vi "System.vi"() -> ()   [LabVIEW 2020]
uses:
  <vilib>/Instr/_visa.llb/VISA Configure Serial Port (Instr).vi
  <vilib>/httpClient/PUTBuffer.vi
  <vilib>/express/express analysis/Spectral/Block/exnSpectralBlock spectral measurements peak poly.vi
  <vilib>/express/express analysis/Spectral/Block/exnSpectralBlock spectral measurements peak DDT.vi
  <vilib>/express/express analysis/Spectral/XNode/ExpressSpectralMeasurementsBlockNode.xnode
  <vilib>/httpClient/LabVIEWHTTPClient.lvlib
panel:
  out "Poor Ventilation":bool
  out "Blade Impact":bool
  out "Normal Operation":bool
  out "?":dbl(knob) scale=0.0..3000.0
  out "Fault 2":dbl
  out "Prediction Started":bool
  out "?":u32
  in  "Current Sensor Threshold":dbl(slide) scale=2.5..2.55
  in  "Arduino COM port":refnum<visa-resource-name>
  out "Vibration Peak":dbl
  out "AI Output":dbl
  out "fft-peak":dbl
  out "data 2":dynamicdata(graph) caption="Sensor Output"
  out "Current Sesnor Output":dbl
  out "?":dbl
  out "?":dbl(knob) scale=0.0..5.0
  out "?":dbl
  out "?":dbl(slide) scale=0.0..100.0
  in  "System stop":bool
  out "?":dbl
  out "FFT":dynamicdata(graph)
  out "Time Domain":dynamicdata(graph)
  # "Fault Detection System For an Industrial Exhaust Fan"
  # "Temperature Sensor"
  # "Current Sensor"
  # "Vibration Sensor"
  # "RPM Sensor"
  # "System Up time (ms)"
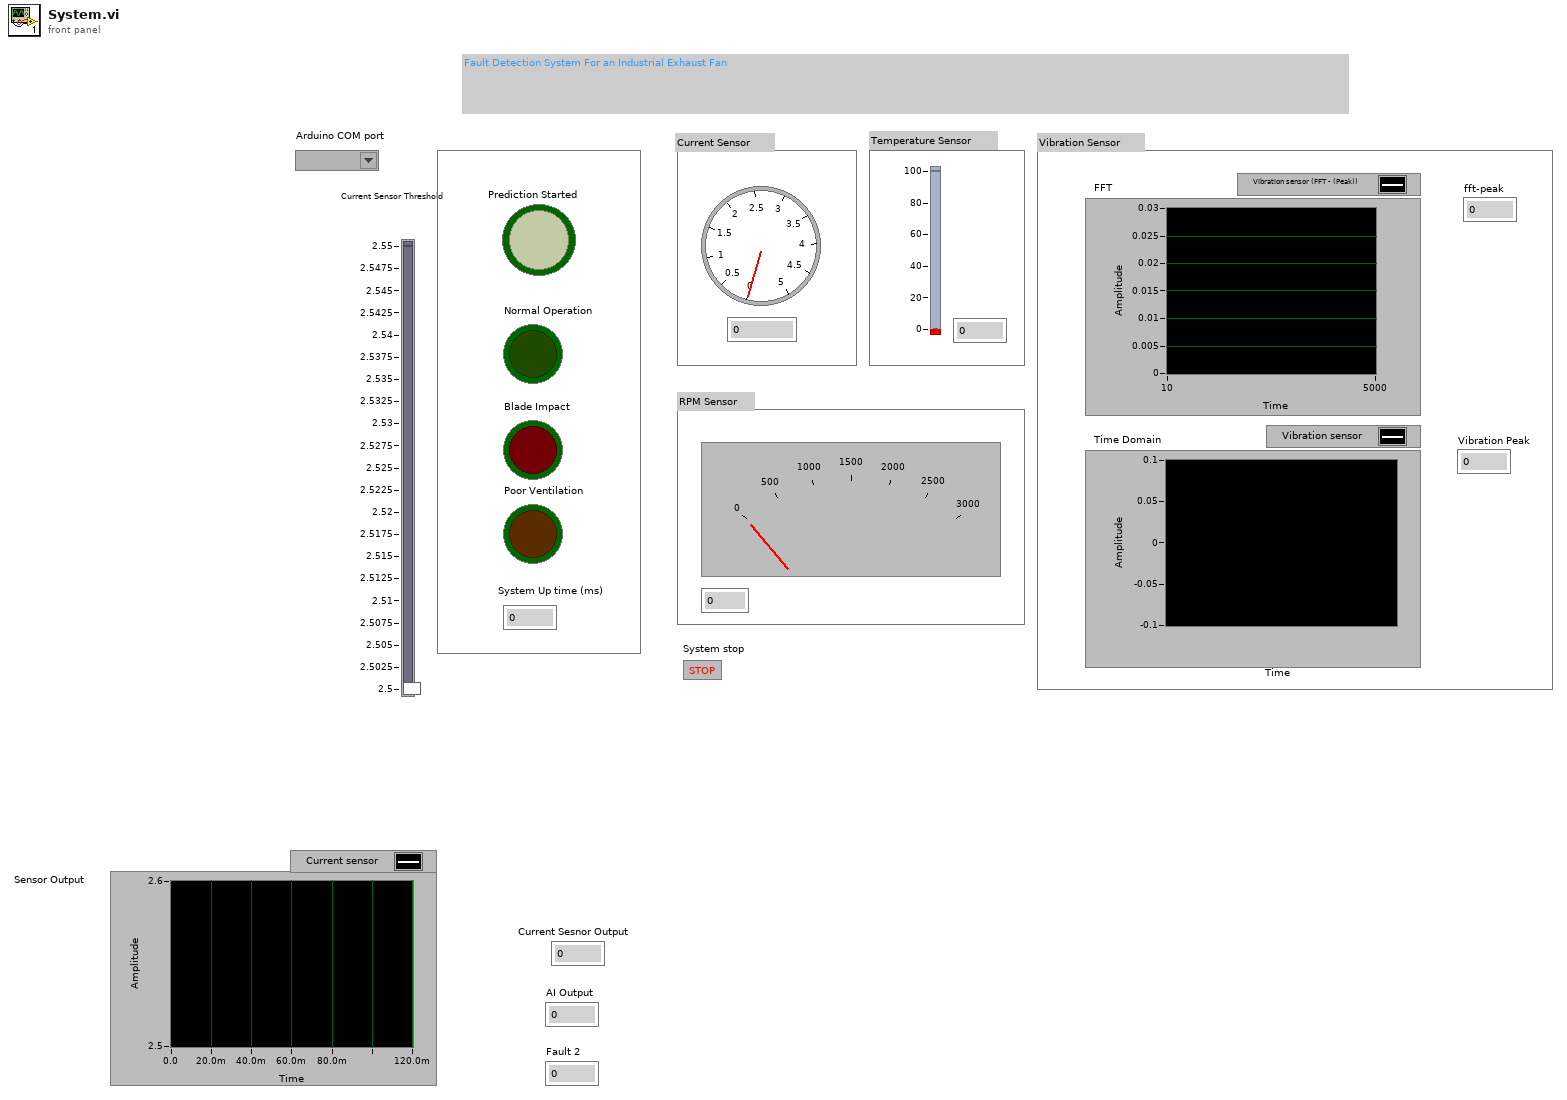
[diagram p1: front panel]
types:
  T1 = cluster{"averaging mode":u16, "weighting mode":u16, "number of averages":u32}
  T2 = cluster{"dB On (F)":bool, "unwrap phase (F)":bool, "convert to degree (F)":bool}
  T3 = typedef "LabVIEWHTTPClient.lvlib/ClientHandle.ctl" = refnum<k1>
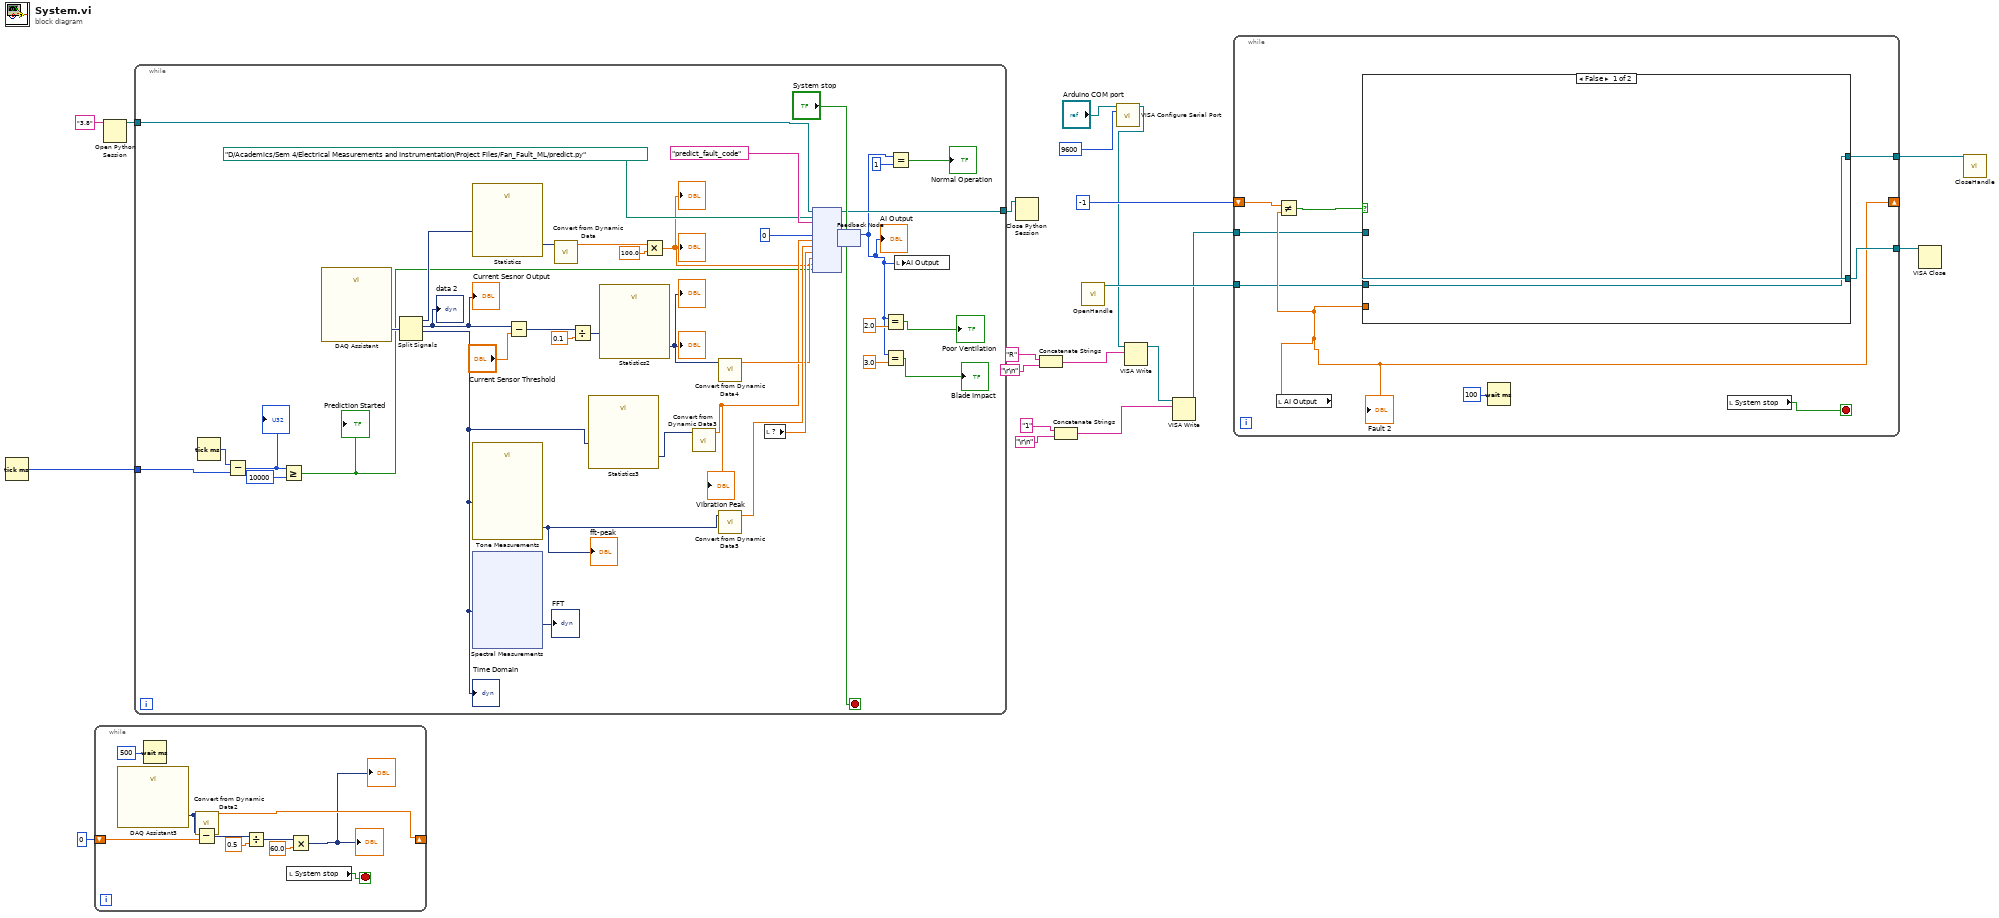
[diagram p0: block diagram]
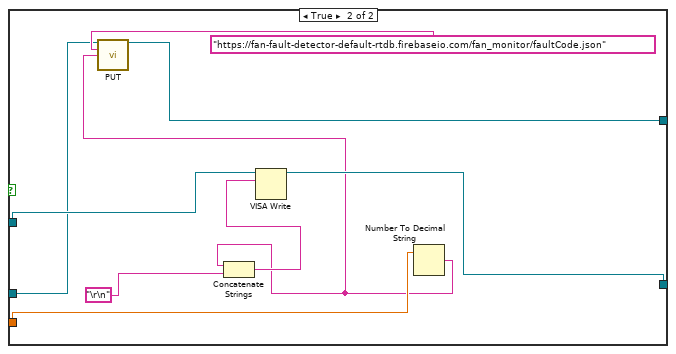
[diagram p2: hidden frame]
diagram:
  n1 = Tick Count (ms)() -> (millisecond timer value=w6:u32)
  n2 = while {
    shift-right: [w28] -> _
    shift-left: 0 -> [w29]
    stop <- w22 stop-if-true
    n3 = call "DAQ Assistant3"() -> ("data"=w23:dynamicdata)  [unwired: 16 in, 3 out]
    n4 = Wait (ms)(milliseconds to wait=u32 500) -> ()  [unwired: 1 out]
    n5 = call "Convert from Dynamic Data2"("Dynamic Data Type"=w23) -> ("Scalar"=w28:dbl)  [unwired: 3 in]
    n6 = Subtract(x=w23, y=w29) -> (x-y=w27:dynamicdata)
    n7 = Divide(x=w27, y=0.5) -> (x/y=w26:dynamicdata)
    n8 = local read "System stop"() -> (w22:bool)
    n9 = Multiply(x=w26, y=60.0) -> (x*y=→"?" →"?":dynamicdata)
  }
  n10 = Open Python Session(python version="3.8" ("Python version")) -> (session out=w18:refnum<k35>)  [unwired: 2 in, 1 out]
  n11 = while {
    tunnel: w18 -> [w51]
    tunnel: [w52] -> w17
    tunnel: w6 -> [w39]
    stop <- "System stop" stop-if-true
    n12 = Tick Count (ms)() -> (millisecond timer value=w42:u32)
    n13 = Subtract(x=w42, y=w39) -> (x-y=w41:u32)
    "?" <- w41
    n14 = Greater Or Equal?(x=w41, y=u32 10000) -> (x >= y?=w38:bool)
    "Prediction Started" <- w38
    n15 = call "DAQ Assistant"() -> ("data"=w63:dynamicdata)  [unwired: 16 in, 3 out]
    n16 = Split Signals(w63) -> (w60:dynamicdata, w62:dynamicdata, w49:dynamicdata)  [unwired: 4 in, 1 out]
    "Time Domain" <- w49
    "Current Sesnor Output" <- w62
    "data 2" <- w62
    n17 = call "Statistics"("Signals"=w60) -> ("Arithmetic Mean"=w68:dynamicdata)  [unwired: 25 in, 1 out]
    n18 = call "Tone Measurements"("Signals"=w49) -> ("Amplitude"=w50:dynamicdata)  [unwired: 8 in, 2 out]
    "fft-peak" <- w50
    n19 = xnode "Spectral Measurements"("Signals"=w49) -> ("FFT - (Peak)"=→"FFT":dynamicdata)  [unwired: 1 in, 2 out]
    n20 = Subtract(x=w62, y="Current Sensor Threshold") -> (x-y=w65:dynamicdata)
    n21 = call "Convert from Dynamic Data"("Dynamic Data Type"=w68) -> ("Scalar"=w67:dbl)  [unwired: 3 in]
    n22 = Divide(x=w65, y=0.1) -> (x/y=w61:dynamicdata)
    n23 = call "Statistics3"("Signals"=w49) -> ("Maximum"=w48:dynamicdata)  [unwired: 25 in, 1 out]
    n24 = call "Statistics2"("Signals"=w61) -> ("Arithmetic Mean"=w59:dynamicdata)  [unwired: 25 in, 1 out]
    "?" <- w59
    "?" <- w59
    n25 = Multiply(x=w67, y=100.0) -> (x*y=w37:dbl)
    "?" <- w37
    "?" <- w37
    n26 = call "Convert from Dynamic Data3"("Dynamic Data Type"=w48) -> ("Scalar"=w47:dbl)  [unwired: 3 in]
    "Vibration Peak" <- w47
    n27 = call "Convert from Dynamic Data4"("Dynamic Data Type"=w59) -> ("Scalar"=w54:dbl)  [unwired: 3 in]
    n28 = call "Convert from Dynamic Data5"("Dynamic Data Type"=w50) -> ("Scalar"=w56:dbl)  [unwired: 3 in]
    n29 = local read item#2() -> (w55:dbl)
    n30 = node ("predict_fault_code")(w51, path "D:/Academics/Sem 4/Electrical Measurements and Instrumentation/Project Files/Fan_Fault_ML/predict.py" ("module path"), "predict_fault_code" ("function name"), 0, w47, w56, w55, w54, w37, w38) -> (w52:refnum<k35>, w32:i32)  [unwired: 7 in, 3 out]
    n31 = feedback-in #1(w32) -> ()
    n32 = feedback #1() -> (w31:i32)  [unwired: 1 in]
    "AI Output" <- w31
    n33 = Equal?(x=w31, y=2.0) -> (x = y?=→"Poor Ventilation":bool)
    n34 = Equal?(x=w31, y=3.0) -> (x = y?=→"Blade Impact":bool)
    n35 = Equal?(x=w31, y=1) -> (x = y?=→"Normal Operation":bool)
    n36 = local write "AI Output"(w31) -> ()
  }
  n37 = Close Python Session(session in=w17) -> ()  [unwired: 1 in, 1 out]
  n38 = Concatenate Strings("R", "\r\n") -> (w8:string)
  n39 = Concatenate Strings("1", "\r\n") -> (w3:string)
  n40 = call <vilib>:"OpenHandle.vi"() -> ("client handle out"=w12:T3)  [unwired: 14 in, 1 out]
  n41 = call-poly "VISA Configure Serial Port"("VISA resource name"="Arduino COM port", "baud rate (9600)"=u32 9600) -> ("VISA resource name out"=w7:refnum<visa-resource-name>)  [unwired: 12 in, 1 out]
  n42 = VISA Write(VISA resource name=w7, write buffer=w8) -> (VISA resource name out=w2:refnum<visa-resource-name>)  [unwired: 1 in, 2 out]
  n43 = VISA Write(VISA resource name=w2, write buffer=w3) -> (VISA resource name out=w1:refnum<visa-resource-name>)  [unwired: 1 in, 2 out]
  n44 = while {
    tunnel: [w88] -> w14
    shift-right: [w83] -> _
    shift-left: -1 -> [w86]
    tunnel: w12 -> [w82]
    tunnel: [w81] -> w11
    tunnel: w1 -> [w80]
    stop <- w85 stop-if-true
    n45 = local read "AI Output"() -> (w83:dbl)
    "Fault 2" <- w83
    n46 = Not Equal?(x=w86, y=w83) -> (x != y?=w87:bool)
    n47 = case shown="False" w87 {
      tunnel: w80 -> [w90 w99]
      tunnel: [w90 w96] -> w88
      tunnel: w83 -> [_ w95]
      tunnel: w82 -> [w89 w93]
      tunnel: [w89 w91] -> w81
      frame False {
      }
      frame True {
        n48 = Number To Decimal String(number=w95) -> (decimal integer string=w92:string)  [unwired: 1 in]
        n49 = call-poly <vilib>:"PUT.vi"("client handle"=w93, "url"="https://fan-fault-detector-default-rtdb.firebaseio.com/fan_monitor/faultCode.json", "buffer"=w92) -> ("client handle out"=w91:T3)  [unwired: 9 in, 3 out]
        n50 = Concatenate Strings(w92, "\r\n") -> (w97:string)
        n51 = VISA Write(VISA resource name=w99, write buffer=w97) -> (VISA resource name out=w96:refnum<visa-resource-name>)  [unwired: 1 in, 2 out]
      }
    }
    n52 = Wait (ms)(milliseconds to wait=u32 100) -> ()  [unwired: 1 out]
    n53 = local read "System stop"() -> (w85:bool)
  }
  n54 = VISA Close(VISA resource name=w14) -> ()  [unwired: 1 in, 1 out]
  n55 = call <vilib>:"CloseHandle.vi"("client handle"=w11) -> ()  [unwired: 14 in, 1 out]
